vi "Get Port Direction.vi"(10 "port":T2) -> (2 "direction":T1)   [LabVIEW 2020, in "AIM ARINC 429 System Explorer.lvlib" / "Implementation.lvlib"]
uses:
  Implementation.lvlib
  Shared/VS Channels Definition for All Labels on Hardware Channel.ctl
  Shared/Direction.ctl
  Shared/VS Channels Definition for Label.ctl
  Shared/VS Channel Definition for Parameter.ctl
  Shared/Parameter Definition.ctl
  <vilib>/NI/NI VeriStand Encoding and Decoding/Encoding.ctl
  Shared/Transfer Type.ctl
  <vilib>/NI/NI VeriStand Encoding and Decoding/Encoding and Decoding.lvlib
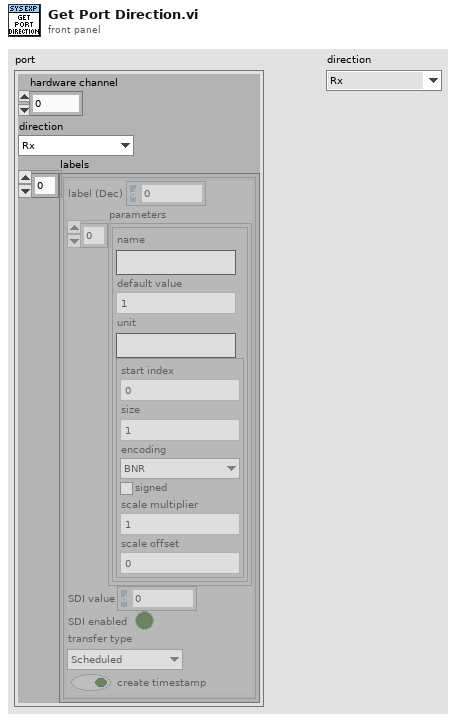
[diagram p1: front panel]
types:
  T1 = typedef "Direction.ctl" = enum16{"Rx", "Tx"}
  T2 = typedef "VS Channels Definition for All Labels on Hardware Channel.ctl" = cluster{"hardware channel":i32, "direction":T1, "labels":T3[]}
  T3 = typedef "VS Channels Definition for Label.ctl" = cluster{"label (Dec)":u32, "parameters":T4[], "SDI value":u8, "SDI enabled":bool, "transfer type":T7, "create timestamp":bool}
  T4 = typedef "VS Channel Definition for Parameter.ctl" = cluster{"name":string, "default value":dbl, "unit":string, "Parameter":T5}
  T5 = typedef "Parameter Definition.ctl" = cluster{"start index":i32, "size":i32, "encoding":T6, "signed":bool, "scale multiplier":dbl, "scale offset":dbl}
  T6 = typedef "Encoding and Decoding.lvlib/Encoding.ctl" = enum16{"BNR", "BCD", "Discrete"}
  T7 = typedef "Transfer Type.ctl" = enum16{"Scheduled", "Acyclic", "Block", "Strobe"}
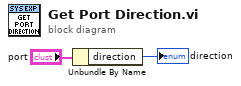
[diagram p0: block diagram]
diagram:
  n1 = Unbundle By Name("port") -> ("direction"=→"direction":T1)
